vi "OSU_Set_Switch.vi"(8 "error in (no error)":errorcluster, 10 "channel":u16, 11 ".NET Reference in":refnum<k24>) -> (0 "error out":errorcluster, 3 "Reference out":refnum<k24>)   [LabVIEW 2017]
uses:
  C:/Users/Ssantec_Test/Documents/Instrument_DLL_Sample_Labview_20250826_Ver1.5.0_x64/DLL/InstrumentDLL.dll
  DLL/InstrumentDLL.dll
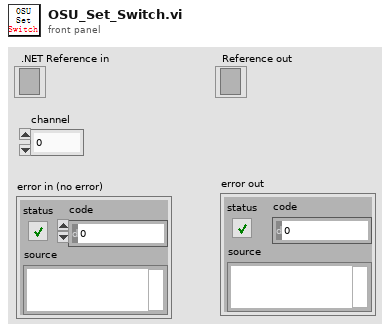
[diagram p1: front panel]
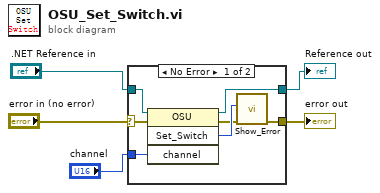
[diagram p0: block diagram]
diagram:
  n1 = case shown="No Error" "error in (no error)" {
    selector: "error in (no error)" -> [w9 w14]
    tunnel: "channel" -> [w12 _]
    tunnel: ".NET Reference in" -> [w11 w13]
    tunnel: [w10 w13] -> w3
    tunnel: [w6 w14] -> w1
    frame No Error {
      n2 = invoke on="调用节点" class="OSU" method="Set_Switch"(reference=w11, error in=w9, "channel"=w12) -> (reference out=w10:refnum<k24>, error out=w7:errorcluster, "Set_Switch"=w8:i32)  [unwired: 1 in, 1 out]
      n3 = call "Show_Error.vi"("error in (no error)"=w7, "Error"=w8) -> ("error out"=w6:errorcluster)  [unwired: 9 in]
    }
    frame Error {
    }
  }
  "error out" <- w1
  "Reference out" <- w3
